vi "Lift.vi"() -> ()   [LabVIEW 2014]
panel:
  out "finish":bool
  out "operating":bool
  out "error":bool
  out "direction 1Down|0Up":dbl
  out "motor":bool
  in  "stop":bool
  in  "User Input":bool[](array[boolean])
  in  "Limit switch":bool[](array[boolean])
  # "Up switch 0"
  # "Down switch 1"
  # "Max Limit switch"
  # "Min Limit switch"
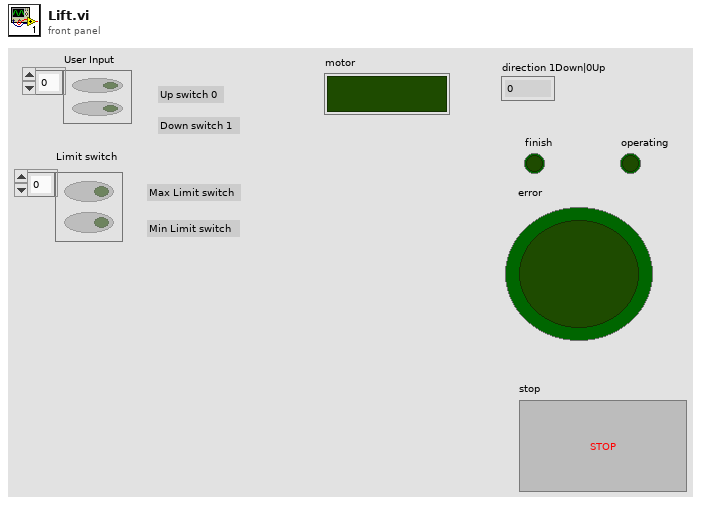
[diagram p1: front panel]
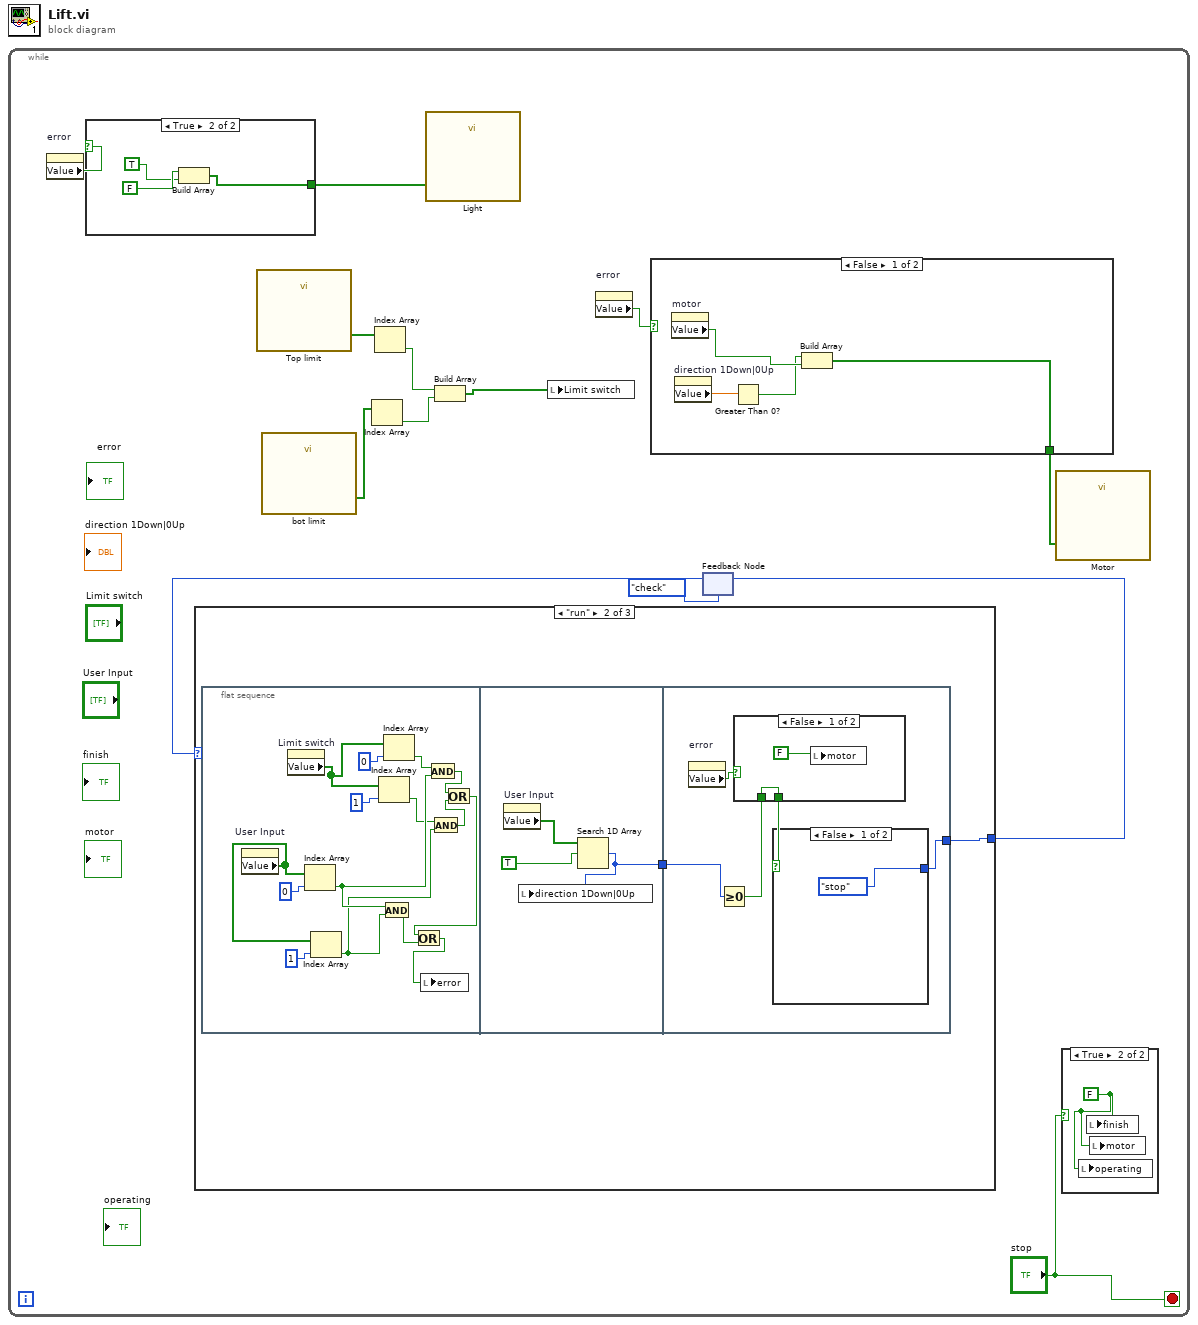
[diagram p0: block diagram]
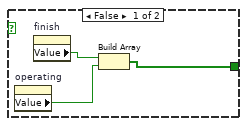
[diagram p3: hidden frame]
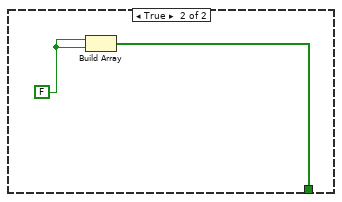
[diagram p4: hidden frame]
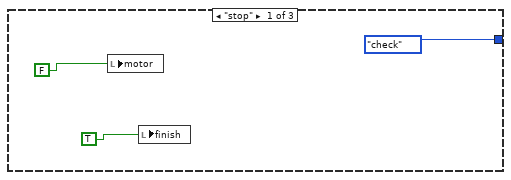
[diagram p5: hidden frame]
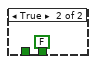
[diagram p6: hidden frame]
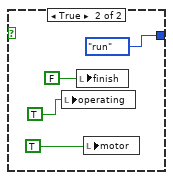
[diagram p7: hidden frame]
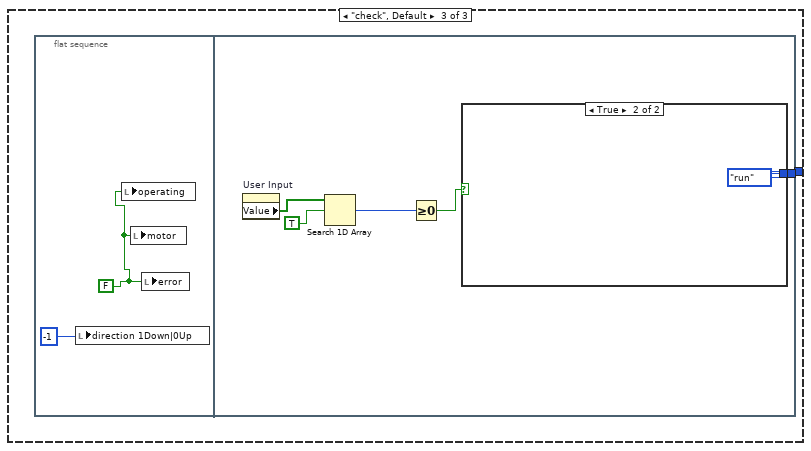
[diagram p8: hidden frame]
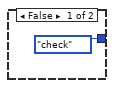
[diagram p9: hidden frame]
diagram:
  n1 = while {
    stop <- "stop" stop-if-true
    n2 = property on="error" class="Bool (strict)"() -> ("Value"=w3:bool)  [unwired: 2 in, 2 out]
    n3 = case shown="True" w3 {
      tunnel: [w15 w20] -> w2
      frame False {
        n4 = property on="operating" class="Bool (strict)"() -> ("Value"=w17:bool)  [unwired: 2 in, 2 out]
        n5 = property on="finish" class="Bool (strict)"() -> ("Value"=w16:bool)  [unwired: 2 in, 2 out]
        n6 = Build Array(w16, w17) -> (w15:bool[])
      }
      frame True {
        n7 = Build Array(FALSE, TRUE) -> (w20:bool[])
      }
    }
    n8 = call "Top limit"() -> ("data"=w8:bool[])  [unwired: 17 in, 2 out]
    n9 = call "bot limit"() -> ("data"=w10:bool[])  [unwired: 17 in, 2 out]
    n10 = Index Array(array=w10) -> (element=w9:bool)  [unwired: 1 in]
    n11 = Index Array(array=w8) -> (element=w7:bool)  [unwired: 1 in]
    n12 = call "Light"("data"=w2) -> ()  [unwired: 17 in, 2 out]
    n13 = Build Array(w7, w9) -> (w6:bool[])
    n14 = local write "Limit switch"(w6) -> ()
    n15 = property on="error" class="Bool (strict)"() -> ("Value"=w4:bool)  [unwired: 2 in, 2 out]
    n16 = case shown="False" w4 {
      tunnel: [w23 w25] -> w5
      frame False {
        n17 = property on="motor" class="Bool (strict)"() -> ("Value"=w22:bool)  [unwired: 2 in, 2 out]
        n18 = property on="direction 1Down|0Up" class="DigNum (strict)"() -> ("Value"=w24:dbl)  [unwired: 2 in, 2 out]
        n19 = Greater Than 0?(x=w24) -> (x > 0?=w21:bool)
        n20 = Build Array(w21, w22) -> (w23:bool[])
      }
      frame True {
        w26 = FALSE
        n21 = Build Array(w26, w26) -> (w25:bool[])
      }
    }
    n22 = feedback #1(enum16{"stop", "run", "check"}."check") -> (w12:enum16{"stop", "run", "check"})
    n23 = case shown="\"run\"" w12 {
      tunnel: [enum16{"stop", "run", "check"}."check" w31 w63] -> w13
      frame "stop" {
        n24 = local write "motor"(FALSE) -> ()
        n25 = local write "finish"(TRUE) -> ()
      }
      frame "run" {
        n26 = flat-sequence {
          tunnel: [w47] -> w30
          tunnel: [w54] -> w31
          tunnel: w30 -> [w53]
          frame #0 {
            n27 = property on="User Input" class="Arr (strict)"() -> ("Value"=w44:bool[])  [unwired: 2 in, 2 out]
            n28 = property on="Limit switch" class="Arr (strict)"() -> ("Value"=w41:bool[])  [unwired: 2 in, 2 out]
            n29 = Index Array(array=w44, index=0) -> (element=w39:bool)
            n30 = Index Array(array=w44, index=1) -> (element=w37:bool)
            n31 = Index Array(array=w41, index=1) -> (element=w38:bool)
            n32 = And(x=w39, y=w37) -> (x .and. y?=w33:bool)
            n33 = Index Array(array=w41, index=0) -> (element=w40:bool)
            n34 = And(x=w40, y=w39) -> (x .and. y?=w36:bool)
            n35 = And(x=w38, y=w37) -> (x .and. y?=w35:bool)
            n36 = Or(x=w36, y=w35) -> (x .or. y?=w34:bool)
            n37 = Or(x=w34, y=w33) -> (x .or. y?=w32:bool)
            n38 = local write "error"(w32) -> ()
          }
          frame #1 {
            n39 = property on="User Input" class="Arr (strict)"() -> ("Value"=w49:bool[])  [unwired: 2 in, 2 out]
            n40 = Search 1D Array(1D array=w49, element=TRUE) -> (index of element=w47:i32)  [unwired: 1 in]
            n41 = local write "direction 1Down|0Up"(w47) -> ()
          }
          frame #2 {
            n42 = property on="error" class="Bool (strict)"() -> ("Value"=w52:bool)  [unwired: 2 in, 2 out]
            n43 = Greater Or Equal To 0?(x=w53) -> (x >= 0?=w50:bool)
            n44 = case shown="False" w52 {
              tunnel: [w56 FALSE] -> w51
              tunnel: w50 -> [w56 _]
              frame False {
                n45 = local write "motor"(FALSE) -> ()
              }
              frame True {
              }
            }
            n46 = case shown="False" w51 {
              tunnel: [enum16{"stop", "run", "check"}."stop" enum16{"stop", "run", "check"}."run"] -> w54
              frame False {
              }
              frame True {
                n47 = local write "operating"(TRUE) -> ()
                n48 = local write "finish"(FALSE) -> ()
                n49 = local write "motor"(TRUE) -> ()
              }
            }
          }
        }
      }
      frame "check", Default {
        n50 = flat-sequence {
          tunnel: [w70] -> w63
          frame #0 {
            w64 = FALSE
            n51 = local write "direction 1Down|0Up"(-1) -> ()
            n52 = local write "operating"(w64) -> ()
            n53 = local write "motor"(w64) -> ()
            n54 = local write "error"(w64) -> ()
          }
          frame #1 {
            n55 = property on="User Input" class="Arr (strict)"() -> ("Value"=w69:bool[])  [unwired: 2 in, 2 out]
            n56 = Search 1D Array(1D array=w69, element=TRUE) -> (index of element=w67:i32)  [unwired: 1 in]
            n57 = Greater Or Equal To 0?(x=w67) -> (x >= 0?=w66:bool)
            n58 = case shown="True" w66 {
              tunnel: [enum16{"stop", "run", "check"}."check" enum16{"stop", "run", "check"}."run"] -> w70
              frame False {
              }
              frame True {
              }
            }
          }
        }
      }
    }
    n59 = feedback-in #1(w13) -> ()
    n60 = call "Motor"("data"=w5) -> ()  [unwired: 17 in, 2 out]
    n61 = case shown="True" "stop" {
      frame False {
      }
      frame True {
        w14 = FALSE
        n62 = local write "operating"(w14) -> ()
        n63 = local write "finish"(w14) -> ()
        n64 = local write "motor"(w14) -> ()
      }
    }
  }
